vi "GBD_FileConvert.vi"() -> ()   [LabVIEW 2017, in "GL860_Driver.lvlib"]
uses:
  GL860_Driver.lvlib
panel:
  in  "ファイル変換":bool
  in  "GBDファイルパス":path
  in  "閉じる":bool
  in  "CSVファイルパス":path
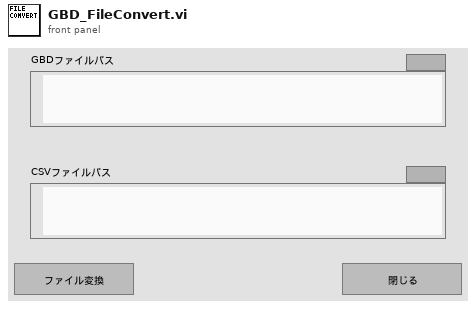
[diagram p1: front panel]
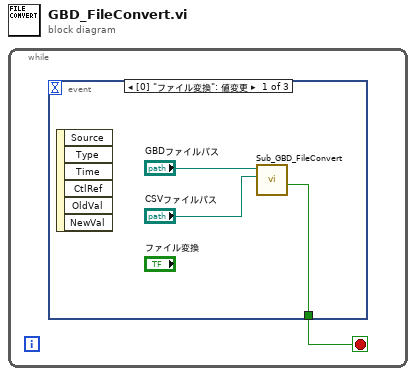
[diagram p0: block diagram]
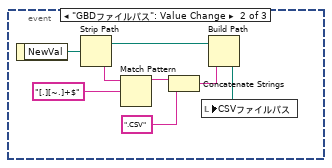
[diagram p2: hidden frame]
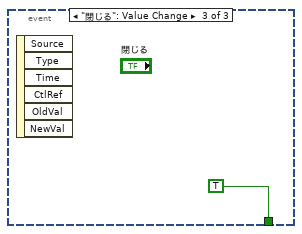
[diagram p3: hidden frame]
diagram:
  n1 = while {
    stop <- w1 stop-if-true
    n2 = event shown="[0] \"ファイル変換\": 値変更" {
      selector: _ -> [_ _ _]
      dyn-events: _ -> [_ _ _]
      timeout: _ -> [_ _ _]
      tunnel: [w2 _ TRUE] -> w1
      event "ファイル変換": Value Change {
        n3 = event-data() -> ()  [unwired: 1 in, 6 out]
        n4 = call "Sub_GBD_FileConvert.vi"("CSV"="CSVファイルパス", "GBD"="GBDファイルパス") -> ("EOF"=w2:bool)  [unwired: 8 in, 1 out]
      }
      event "GBDファイルパス": Value Change {
        n5 = event-data() -> ("NewVal"=w12:path)  [unwired: 1 in]
        n6 = Strip Path(path=w12) -> (stripped path=w11:path, name=w10:string)
        n7 = Match Pattern(string=w10, regular expression="[.][~.]+$") -> (before substring=w8:string)  [unwired: 1 in, 3 out]
        n8 = Concatenate Strings(w8, ".CSV" ("regular expression")) -> (w6:string)
        n9 = Build Path(base path=w11, name or relative path=w6) -> (appended path=w5:path)
        n10 = local write "CSVファイルパス"(w5) -> ()
      }
      event "閉じる": Value Change {
        n11 = event-data() -> ()  [unwired: 1 in, 6 out]
      }
    }
  }
